vi "SLL DE DAQ Info Display.vi"(8 "error in (no error)":errorcluster) -> (0 "error out":errorcluster)   [LabVIEW 2013]
doc: "Copyright © 2005, Soliton Technologies.\nAll rights reserved."
uses:
  Controls/SLL DE DAQ Info Display Options.ctl
  Sub VIs/DAQ Engine/Controls/SLL DE DI Global Options.ctl
  Sub VIs/DAQ Engine/Controls/SLL DE Circular Buffer Options.ctl
  Sub VIs/DAQ Engine/Controls/SLL DE DO Global Options.ctl
  Sub VIs/DAQ Engine/Controls/SLL DE AO Global Options.ctl
  Sub VIs/DAQ Engine/Controls/SLL DE DAQ Global Options.ctl
  Sub VIs/DAQ Engine/Controls/SLL DE DAQ Global Elements.ctl
  Sub VIs/DAQ Engine/Controls/SLL DE List of Digital Inputs.ctl
  Sub VIs/DAQ Engine/Controls/SLL DE List of Analog Inputs.ctl
  Sub VIs/DAQ Engine/Controls/SLL DE List of Digital Outputs.ctl
  Sub VIs/DAQ Engine/Controls/SLL DE List of Analog Outputs.ctl
panel:
  in  "View File":bool
  in  "Virtual Chart":bool
  out "DO Running?":bool
  out "DI Running?":bool
  out "AO Running?":bool
  out "AI Running?":bool
  in  "List of Analog Outputs":T1
  in  "stop":bool
  in  "Tab Control":T2(tab)
  out "AI Status 3":cluster{"AI Value":sgl, "AI Name":string}[](array[cluster]) {"AI Value" format="%#.2f"}
  out "AI Status 2":cluster{"AI Value":sgl, "AI Name":string}[](array[cluster]) {"AI Value" format="%#.2f"}
  out "AI Status":cluster{"AI Value":sgl, "AI Name":string}[](array[cluster]) {"AI Value" format="%#.2f"}
  in  "AO Status":cluster{"AO Value":sgl, "AO Name":string}[](array[cluster]) {"AO Value" format="%#.2f"}
  in  "AO Status 2":cluster{"AO Value":sgl, "AO Name":string}[](array[cluster]) {"AO Value" format="%#.2f"}
  in  "AO Status 3":cluster{"AO Value":sgl, "AO Name":string}[](array[cluster]) {"AO Value" format="%#.2f"}
  out "DI Status 3":cluster{"DI Value?":bool, "DI Name":string}[](array[cluster])
  out "DI Status 2":cluster{"DI Value?":bool, "DI Name":string}[](array[cluster])
  out "DI Status":cluster{"DI Value?":bool, "DI Name":string}[](array[cluster])
  in  "DO Status 3":string[](array[string])
  in  "DO Value? 3":bool[](array[boolean]) caption="DO Value?"
  in  "DO Status 2":string[](array[string])
  in  "DO Value? 2":bool[](array[boolean]) caption="DO Value?"
  in  "DO Status":string[](array[string])
  in  "DO Value?":bool[](array[boolean]) caption="Enable Test"
  out "Date":string="Fri, Oct 10, 2003 3:32:43 AM"
  in  "List of Digital Outputs":T3=enum."STATION1_STOP TEST"
  in  "List of Analog Inputs":T4
  in  "List of Digital Inputs":T5
  # "<Project Name>"
  # "Logo"
  # "DAQ Info Display SCREEN"
  # "="
  # "="
  # "="
  # "-"
  # "-"
  # "-"
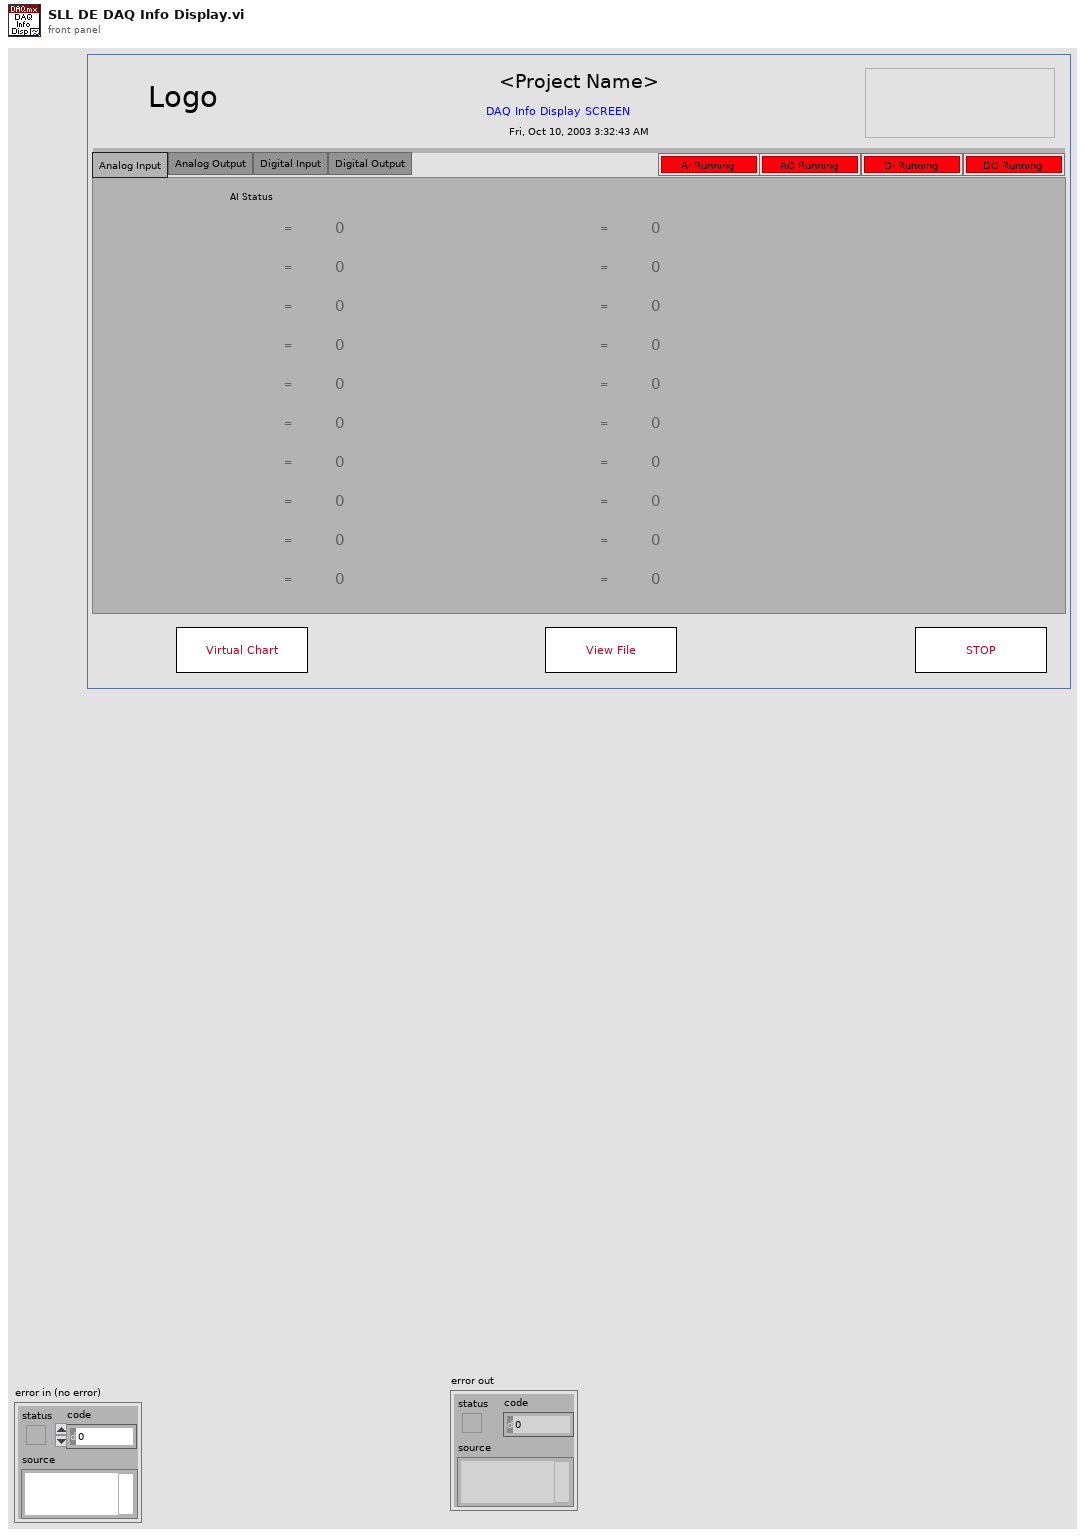
[diagram p1: front panel]
types:
  T1 = typedef "SLL DE List of Analog Outputs.ctl" = enum16{"None"}
  T2 = enum32{"Analog Input", "Analog Output", "Digital Input", "Digital Output"}
  T3 = typedef "SLL DE List of Digital Outputs.ctl" = enum16{"STATION1_START TEST", "STATION1_STOP TEST", "STATION1_LIGHT1", "STATION1_LIGHT2", "STATION1_LIGHT3", "STATION1_SELECT_TEST", "STATION2_START TEST", "STATION2_STOP TEST", "STATION2_LIGHT1", "STATION2_LIGHT2", "STATION2_LIGHT3", "STATION2_SELECT_TEST", "STATION3_START TEST", "STATION3_STOP TEST", "STATION3_LIGHT1", "STATION3_LIGHT2", "STATION3_LIGHT3", "STATION3_SELECT_TEST", "STATION4_START TEST", "STATION4_STOP TEST", "STATION4_LIGHT1", "STATION4_LIGHT2", "STATION4_LIGHT3", "STATION4_SELECT_TEST"}
  T4 = typedef "SLL DE List of Analog Inputs.ctl" = enum16{"None"}
  T5 = typedef "SLL DE List of Digital Inputs.ctl" = enum16{"STATION1_START", "STATION1_STOP", "STATION1_CLAMPED", "STATION1_TC_PASS", "STATION1_TC_FAIL", "STATION1_TTA", "STATION1_TTB", "STATION2_START", "STATION2_STOP", "STATION2_CLAMPED", "STATION2_TC_PASS", "STATION2_TC_FAIL", "STATION2_TTA", "STATION2_TTB", "STATION3_START", "STATION3_STOP", "STATION3_CLAMPED", "STATION3_TC_PASS", "STATION3_TC_FAIL", "STATION3_TTA", "STATION3_TTB", "STATION4_START", "STATION4_STOP", "STATION4_CLAMPED", "STATION4_TC_PASS", "STATION4_TC_FAIL", "STATION4_TTA", "STATION4_TTB"}
  T6 = typedef "SLL DE DAQ Info Display Options.ctl" = enum16{"Initialization", "Config AI/DI Controls", "Config AO Controls", "Config DO Controls", "Poll Events", "AI Read", "DI Read", "AO Write", "DO Write", "Launch Virtual Chart", "Launch File View", "Error", "Exit"}
  T7 = cluster{"DI Channel Names":string[], "DI Status":cluster{"DI ON?":bool, "DI Name":string}[], "AI Status":cluster{"AI Value":sgl, "AI Name":string}[], "DO Status":string[], "DO Value?":bool[], "AO Status":cluster{"AI Value":sgl, "AI Name":string}[]}
  T8 = typedef "SLL DE DO Global Options.ctl" = enum16{"Init", "Write Line", "Write Array", "Write Full Status", "Read Line", "Read Array", "Read Full Status", "Restart DO", "Send to Safe Mode", "Stop DO"}
  T9 = typedef "SLL DE AO Global Options.ctl" = enum16{"Init", "Write Line", "Write Array", "Read Line", "Read Array", "Read Full Status", "Restart AO", "Send to Safe Mode", "Stop AO"}
  T10 = typedef "SLL DE DAQ Global Options.ctl" = enum16{"Init", "Write 1", "Read 1", "Write Array", "Read Array", "Clear"}
  T11 = typedef "SLL DE Circular Buffer Options.ctl" = enum16{"Initialize", "Init Pointer X", "Write", "Read Single Value", "Read Pointer X (Multi Value)", "Clear Data"}
  T12 = typedef "SLL DE DI Global Options.ctl" = enum16{"Init", "Write Line", "Write Array", "Read Line", "Read Array", "Read Full Status", "Write Full Status"}
  T13 = typedef "SLL DE DAQ Global Elements.ctl" = enum16{"AI Error", "AO Error", "DI Error", "DO Error", "AI Restart", "DI Restart", "AI Running", "AO Running", "DI Running", "DO Running", "DAQ Exit?"}
  T14 = enum32{"Bad", "Idle", "Run top level", "Running"}
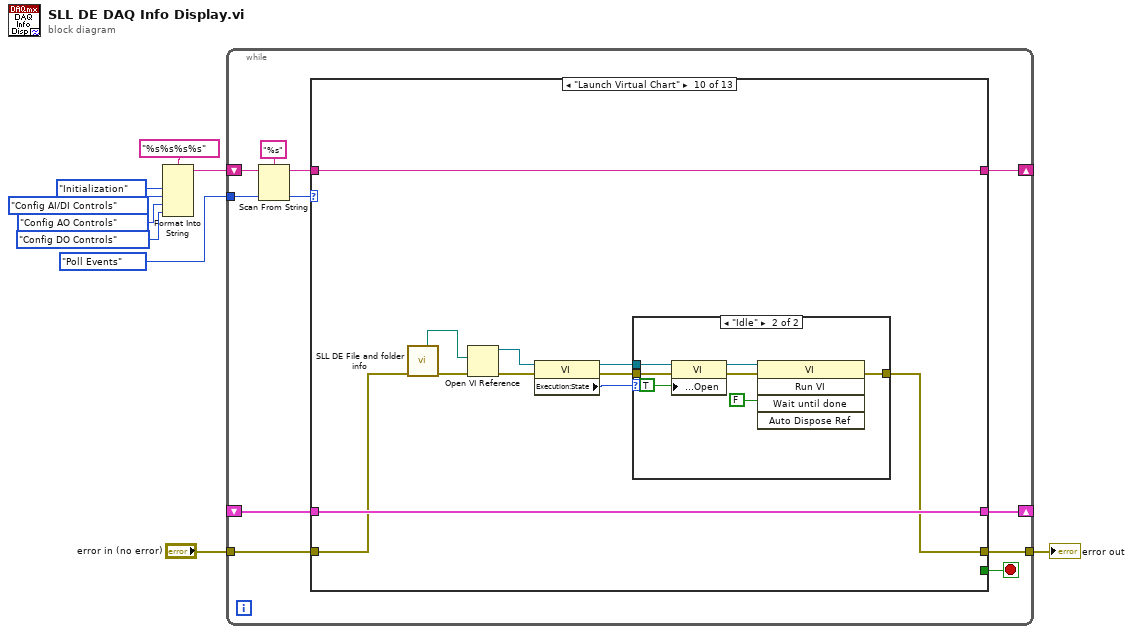
[diagram p0: block diagram]
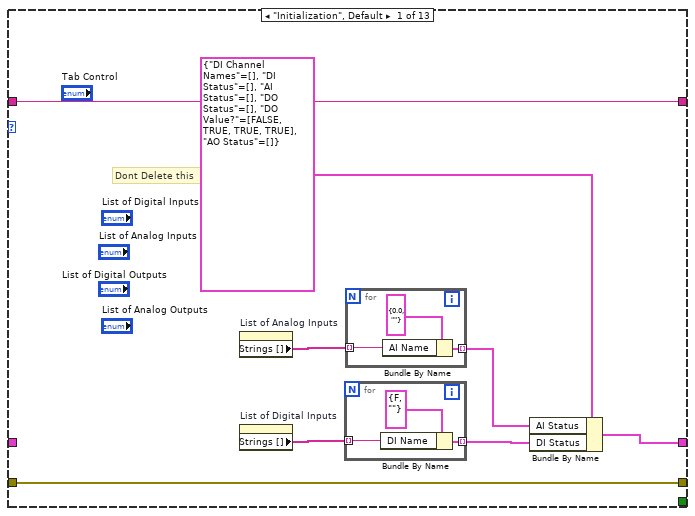
[diagram p2: hidden frame]
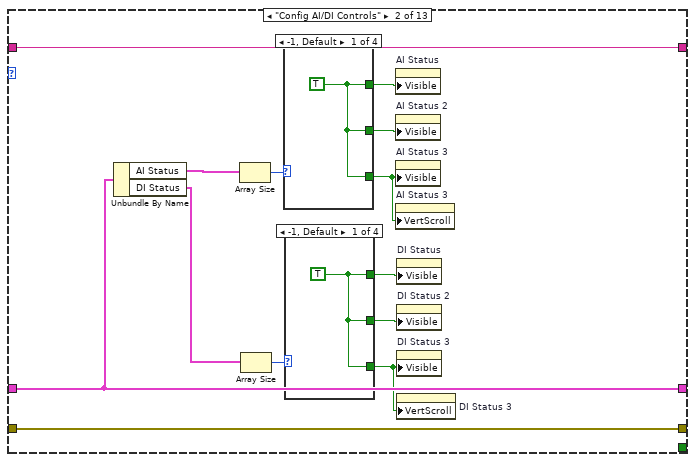
[diagram p3: hidden frame]
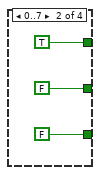
[diagram p4: hidden frame]
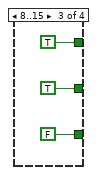
[diagram p5: hidden frame]
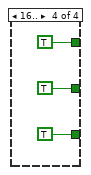
[diagram p6: hidden frame]
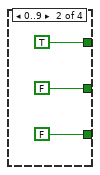
[diagram p7: hidden frame]
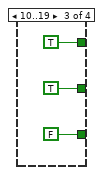
[diagram p8: hidden frame]
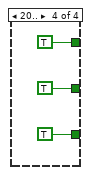
[diagram p9: hidden frame]
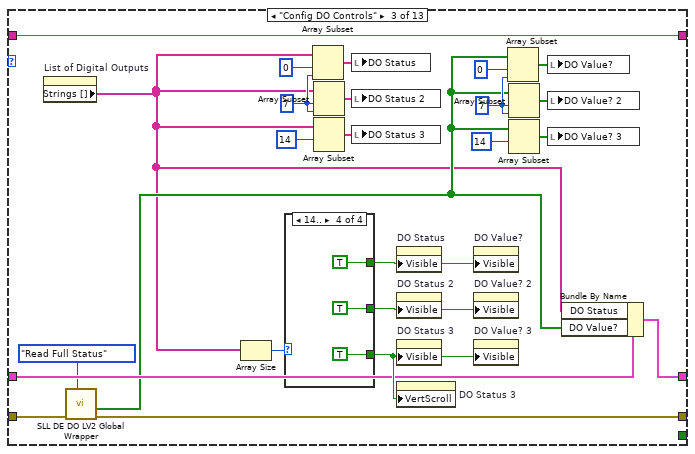
[diagram p10: hidden frame]
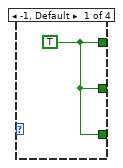
[diagram p11: hidden frame]
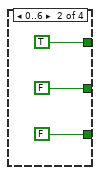
[diagram p12: hidden frame]
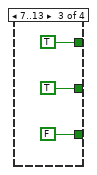
[diagram p13: hidden frame]
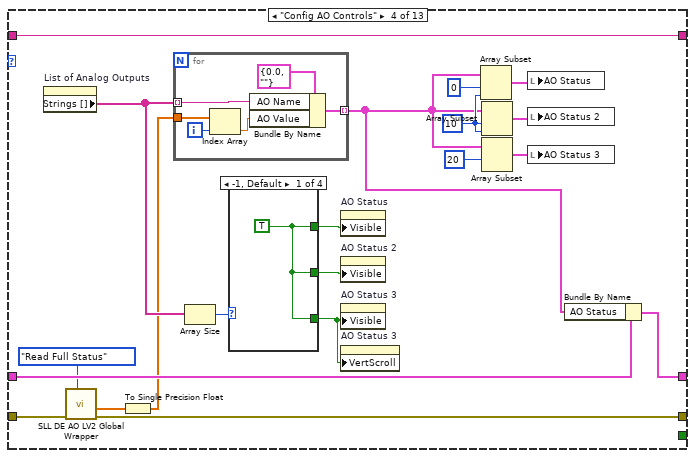
[diagram p14: hidden frame]
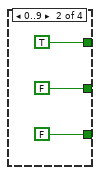
[diagram p15: hidden frame]
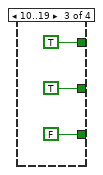
[diagram p16: hidden frame]
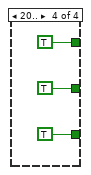
[diagram p17: hidden frame]
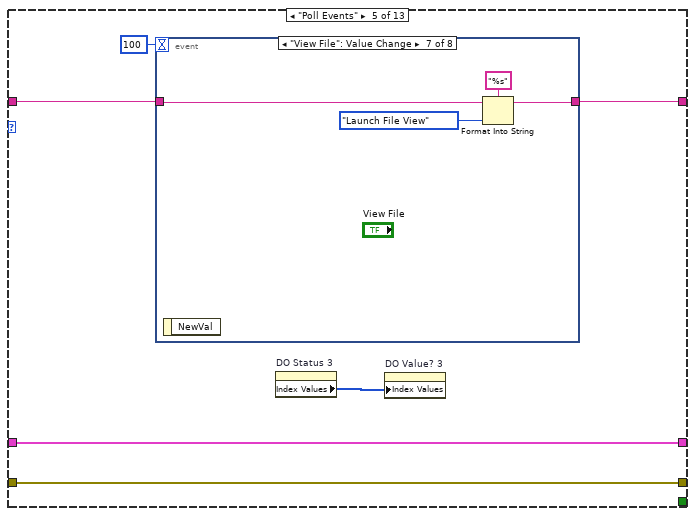
[diagram p18: hidden frame]
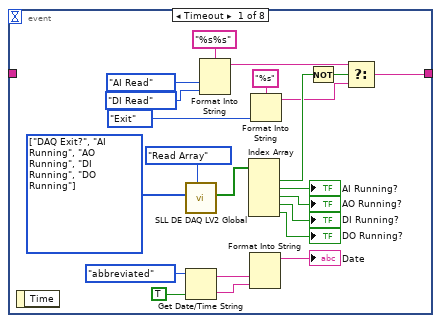
[diagram p19: hidden frame]
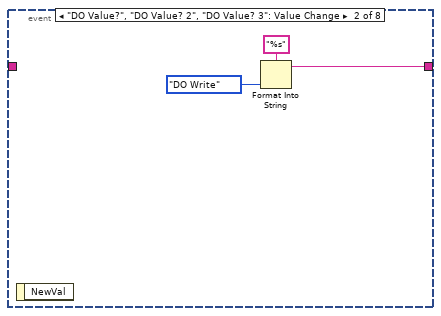
[diagram p20: hidden frame]
diagram:
  n1 = Format Into String(format string="%s%s%s%s", SLL_DE_DAQ_Info_Display_Options."Initialization" ("Case"), SLL_DE_DAQ_Info_Display_Options."Config AI/DI Controls" ("Case"), SLL_DE_DAQ_Info_Display_Options."Config AO Controls" ("Case"), SLL_DE_DAQ_Info_Display_Options."Config DO Controls" ("Case")) -> (resulting string=w8:string)  [unwired: 2 in, 1 out]
  n2 = while {
    shift-right: [w16] -> _
    shift-left: w8 -> [w20]
    tunnel: SLL_DE_DAQ_Info_Display_Options."Poll Events" ("Case") -> [w18]
    tunnel: [w14] -> w5
    tunnel: "error in (no error)" -> [w13]
    shift-right: [w11] -> _
    shift-left: _ -> [w10]
    stop <- w12 stop-if-true
    n3 = Scan From String(format string="%s", input string=w20, default 1=w18) -> (remaining string=w15:string, output 1=w17:T6)  [unwired: 2 in, 2 out]
    n4 = case shown="\"Launch Virtual Chart\"" w17 {
      tunnel: [w28 w44 w91 w121 w140 w229 w250 w270 w297 w308 w327 w338 w342] -> w16
      tunnel: w15 -> [w28 w44 w91 w121 w141 w229 w250 w270 w297 w308 w327 w338 w342]
      tunnel: [w21 w46 w76 w108 w143 w224 w248 w260 w293 w298 w318 w337 w341] -> w14
      tunnel: w13 -> [w21 w46 w77 w109 w143 w225 w249 w261 w294 w306 w325 w337 w341]
      tunnel: [_ _ _ _ _ _ _ _ _ _ _ _ TRUE] -> w12
      tunnel: [w25 w45 w85 w115 w142 w226 w246 w269 w296 w307 w326 w336 w339] -> w11
      tunnel: w10 -> [_ w45 w86 w116 w142 w226 w246 w269 w296 w307 w326 w336 w339]
      frame "Initialization", Default {
        # "Dont Delete this"
        n5 = property on="List of Analog Inputs" class="Enum (strict)"() -> ("Strings []"=w22:string[])  [unwired: 2 in, 2 out]
        n6 = property on="List of Digital Inputs" class="Enum (strict)"() -> ("Strings []"=w27:string[])  [unwired: 2 in, 2 out]
        n7 = for {
          tunnel: w27 -> [w33] mode=indexing
          tunnel: [w32] -> w24 mode=indexing
          n8 = Bundle By Name(cluster=cluster{"DI ON?":bool, "DI Name":string} {"DI ON?"=FALSE, "DI Name"=""} ("Filter Status 2"), "DI Name"=w33) -> (w32:cluster{"DI ON?":bool, "DI Name":string})
        }
        n9 = for {
          tunnel: w22 -> [w31] mode=indexing
          tunnel: [w30] -> w23 mode=indexing
          n10 = Bundle By Name(cluster=cluster{"AI Value":sgl, "AI Name":string} {"AI Value"=0.0, "AI Name"=""} ("Filter Status 2"), "AI Name"=w31) -> (w30:cluster{"AI Value":sgl, "AI Name":string})
        }
        n11 = Bundle By Name(cluster=T7 {"DI Channel Names"=[], "DI Status"=[], "AI Status"=[], "DO Status"=[], "DO Value?"=[FALSE, TRUE, TRUE, TRUE], "AO Status"=[]}, "AI Status"=w23, "DI Status"=w24) -> (w25:T7)
      }
      frame "Config AI/DI Controls" {
        n12 = Unbundle By Name(w45) -> ("AI Status"=w47:cluster{"AI Value":sgl, "AI Name":string}[], "DI Status"=w35:cluster{"DI ON?":bool, "DI Name":string}[])
        n13 = Array Size(array=w47) -> (size(s)=w43:i32)
        n14 = Array Size(array=w35) -> (size(s)=w36:i32)
        n15 = case shown="-1, Default" w43 {
          tunnel: [w58 TRUE ("Visible") TRUE ("Visible") TRUE ("Visible")] -> w42
          tunnel: [w58 FALSE ("Visible") TRUE ("Visible") TRUE ("Visible")] -> w41
          tunnel: [w58 FALSE ("Visible") FALSE ("Visible") TRUE ("Visible")] -> w40
          frame -1, Default {
            w58 = TRUE ("Visible")
          }
          frame 0..9 {
          }
          frame 10..19 {
          }
          frame 20.. {
          }
        }
        n16 = case shown="-1, Default" w36 {
          tunnel: [w48 TRUE ("Visible") TRUE ("Visible") TRUE ("Visible")] -> w37
          tunnel: [w48 FALSE ("Visible") TRUE ("Visible") TRUE ("Visible")] -> w38
          tunnel: [w48 FALSE ("Visible") FALSE ("Visible") TRUE ("Visible")] -> w39
          frame -1, Default {
            w48 = TRUE ("Visible")
          }
          frame 0..7 {
          }
          frame 8..15 {
          }
          frame 16.. {
          }
        }
        n17 = property on="AI Status" class="Arr (strict)"("Visible"=w42) -> ()  [unwired: 2 in, 2 out]
        n18 = property on="AI Status 2" class="Arr (strict)"("Visible"=w41) -> ()  [unwired: 2 in, 2 out]
        n19 = property on="AI Status 3" class="Arr (strict)"("Visible"=w40) -> ()  [unwired: 2 in, 2 out]
        n20 = property on="AI Status 3" class="Arr (strict)"("VertScroll"=w40) -> ()  [unwired: 2 in, 2 out]
        n21 = property on="DI Status" class="Arr (strict)"("Visible"=w37) -> ()  [unwired: 2 in, 2 out]
        n22 = property on="DI Status 2" class="Arr (strict)"("Visible"=w38) -> ()  [unwired: 2 in, 2 out]
        n23 = property on="DI Status 3" class="Arr (strict)"("Visible"=w39) -> ()  [unwired: 2 in, 2 out]
        n24 = property on="DI Status 3" class="Arr (strict)"("VertScroll"=w39) -> ()  [unwired: 2 in, 2 out]
      }
      frame "Config DO Controls" {
        w74 = 7 ("length")
        w83 = 7 ("length")
        n25 = property on="List of Digital Outputs" class="Enum (strict)"() -> ("Strings []"=w68:string[])  [unwired: 2 in, 2 out]
        n26 = call "SLL DE DO LV2 Global Wrapper.vi"("DO Option"=SLL_DE_DO_Global_Options."Read Full Status", "error in (no error)"=w77) -> ("error out"=w76:errorcluster, "Digital Output Array Value"=w69:bool[])  [unwired: 6 in, 2 out]
        n27 = Array Size(array=w68) -> (size(s)=w90:i32)
        n28 = case shown="14.." w90 {
          tunnel: [w92 TRUE ("Visible") TRUE ("Visible") TRUE ("Visible")] -> w87
          tunnel: [w92 FALSE ("Visible") TRUE ("Visible") TRUE ("Visible")] -> w88
          tunnel: [w92 FALSE ("Visible") FALSE ("Visible") TRUE ("Visible")] -> w89
          frame -1, Default {
            w92 = TRUE ("Visible")
          }
          frame 0..6 {
          }
          frame 7..13 {
          }
          frame 14.. {
          }
        }
        n29 = Array Subset(array=w68, index=0, length=w83) -> (w81:string[])
        n30 = Array Subset(array=w68, index=w83, length=w83) -> (w80:string[])
        n31 = Array Subset(array=w68, index=14) -> (w79:string[])  [unwired: 1 in]
        n32 = local write "DO Status"(w81) -> ()
        n33 = local write "DO Status 2"(w80) -> ()
        n34 = local write "DO Status 3"(w79) -> ()
        n35 = property on="DO Status" class="Arr (strict)"("Visible"=w87) -> ()  [unwired: 2 in, 2 out]
        n36 = property on="DO Status 2" class="Arr (strict)"("Visible"=w88) -> ()  [unwired: 2 in, 2 out]
        n37 = property on="DO Status 3" class="Arr (strict)"("Visible"=w89) -> ()  [unwired: 2 in, 2 out]
        n38 = property on="DO Status 3" class="Arr (strict)"("VertScroll"=w89) -> ()  [unwired: 2 in, 2 out]
        n39 = property on="DO Value?" class="Arr (strict)"("Visible"=w87) -> ()  [unwired: 2 in, 2 out]
        n40 = property on="DO Value? 2" class="Arr (strict)"("Visible"=w88) -> ()  [unwired: 2 in, 2 out]
        n41 = property on="DO Value? 3" class="Arr (strict)"("Visible"=w89) -> ()  [unwired: 2 in, 2 out]
        n42 = Array Subset(array=w69, index=0, length=w74) -> (w72:bool[])
        n43 = Array Subset(array=w69, index=w74, length=w74) -> (w71:bool[])
        n44 = Array Subset(array=w69, index=14) -> (w70:bool[])  [unwired: 1 in]
        n45 = local write "DO Value?"(w72) -> ()
        n46 = local write "DO Value? 2"(w71) -> ()
        n47 = local write "DO Value? 3"(w70) -> ()
        n48 = Bundle By Name(cluster=w86, "DO Status"=w68, "DO Value?"=w69) -> (w85:T7)
      }
      frame "Config AO Controls" {
        w113 = 10 ("length")
        n49 = property on="List of Analog Outputs" class="Enum (strict)"() -> ("Strings []"=w111:string[])  [unwired: 2 in, 2 out]
        n50 = call "SLL DE AO LV2 Global Wrapper.vi"("AO Option"=SLL_DE_AO_Global_Options."Read Full Status", "error in (no error)"=w109) -> ("error out"=w108:errorcluster, "Analog Output Array Value"=w106:dbl[])  [unwired: 6 in, 2 out]
        n51 = To Single Precision Float(number=w106) -> (single precision float=w102:sgl[])
        n52 = for {
          tunnel: w111 -> [w127] mode=indexing
          tunnel: [w126] -> w110 mode=indexing
          tunnel: w102 -> [w124]
          i -> [w122]
          n53 = Index Array(array=w124, index=w122) -> (element=w123:sgl)
          n54 = Bundle By Name(cluster=cluster{"AO Value":sgl, "AO Name":string} {"AO Value"=0.0, "AO Name"=""} ("Filter Status 2"), "AO Name"=w127, "AO Value"=w123) -> (w126:cluster{"AO Value":sgl, "AO Name":string})
        }
        n55 = Array Size(array=w111) -> (size(s)=w120:i32)
        n56 = case shown="-1, Default" w120 {
          tunnel: [w128 TRUE ("Visible") TRUE ("Visible") TRUE ("Visible")] -> w117
          tunnel: [w128 FALSE ("Visible") TRUE ("Visible") TRUE ("Visible")] -> w118
          tunnel: [w128 FALSE ("Visible") FALSE ("Visible") TRUE ("Visible")] -> w119
          frame -1, Default {
            w128 = TRUE ("Visible")
          }
          frame 0..9 {
          }
          frame 10..19 {
          }
          frame 20.. {
          }
        }
        n57 = property on="AO Status" class="Arr (strict)"("Visible"=w117) -> ()  [unwired: 2 in, 2 out]
        n58 = property on="AO Status 2" class="Arr (strict)"("Visible"=w118) -> ()  [unwired: 2 in, 2 out]
        n59 = property on="AO Status 3" class="Arr (strict)"("Visible"=w119) -> ()  [unwired: 2 in, 2 out]
        n60 = property on="AO Status 3" class="Arr (strict)"("VertScroll"=w119) -> ()  [unwired: 2 in, 2 out]
        n61 = Array Subset(array=w110, index=0, length=w113) -> (w105:cluster{"AO Value":sgl, "AO Name":string}[])
        n62 = Array Subset(array=w110, index=w113, length=w113) -> (w104:cluster{"AO Value":sgl, "AO Name":string}[])
        n63 = Array Subset(array=w110, index=20) -> (w103:cluster{"AO Value":sgl, "AO Name":string}[])  [unwired: 1 in]
        n64 = local write "AO Status"(w105) -> ()
        n65 = local write "AO Status 2"(w104) -> ()
        n66 = local write "AO Status 3"(w103) -> ()
        n67 = Bundle By Name(cluster=w116, "AO Status"=w110) -> (w115:T7)
      }
      frame "Poll Events" {
        n68 = event shown="[6] \"View File\": Value Change" {
          selector: _ -> [_ _ _ _ _ _ _ _]
          dyn-events: _ -> [_ _ _ _ _ _ _ _]
          timeout: 100 -> [_ _ _ _ _ _ _ _]
          tunnel: w141 -> [_ _ w174 w186 w198 w205 w209 _]
          tunnel: [w148 w166 w175 w187 w199 w206 w210 w213] -> w140
          event Timeout {
            w156 = T13[] [enum."DAQ Exit?", enum."AI Running", enum."AO Running", enum."DI Running", enum."DO Running"] items=["AI Error", "AO Error", "DI Error", "DO Error", "AI Restart", "DI Restart", "AI Running", "AO Running", "DI Running", "DO Running", "DAQ Exit?"] ("Elements Array")
            n69 = event-data() -> ()  [unwired: 1 in, 1 out]
            n70 = call "SLL DE DAQ LV2 Global.vi"("Option"=SLL_DE_DAQ_Global_Options."Read Array", "Elements Array"=w156) -> ("Status Array Out"=w155:bool[])  [unwired: 7 in, 2 out]
            n71 = Get Date/Time String(date format (0)=enum16{"short", "long", "abbreviated"}."abbreviated", want seconds? (F)=TRUE) -> (date string=w160:string, time string=w159:string)  [unwired: 1 in]
            n72 = Format Into String(format string="%s%s", SLL_DE_DAQ_Info_Display_Options."AI Read" ("Case"), SLL_DE_DAQ_Info_Display_Options."DI Read" ("Case")) -> (resulting string=w149:string)  [unwired: 2 in, 1 out]
            n73 = Index Array(array=w155) -> (element #1=w150:bool, element #2=→"AI Running?":bool, element #3=→"AO Running?":bool, element #4=→"DI Running?":bool, element #5=→"DO Running?":bool)  [unwired: 5 in]
            n74 = Format Into String(w160, w159) -> (resulting string=→"Date":string)  [unwired: 3 in, 1 out]
            n75 = Format Into String(format string="%s", SLL_DE_DAQ_Info_Display_Options."Exit" ("Case")) -> (resulting string=w145:string)  [unwired: 2 in, 1 out]
            n76 = Not(x=w150) -> (.not. x?=w144:bool)
            n77 = Select(t=w149, s=w144, f=w145) -> (s? t:f=w148:string)
          }
          event "DO Value?", "DO Value? 2", "DO Value? 3": Value Change {
            n78 = event-data() -> ()  [unwired: 1 in, 1 out]
            n79 = Format Into String(format string="%s", SLL_DE_DAQ_Info_Display_Options."DO Write" ("Case")) -> (resulting string=w166:string)  [unwired: 2 in, 1 out]
          }
          event "AO Status": Value Change {
            n80 = event-data() -> ("NewVal"=w173:cluster{"AO Value":sgl, "AO Name":string}[], "OldVal"=w172:cluster{"AO Value":sgl, "AO Name":string}[])  [unwired: 1 in]
            n81 = Array Size(array=w173) -> (size(s)=w171:i32)
            n82 = Array Size(array=w172) -> (size(s)=w169:i32)
            n83 = Not Equal?(x=w171, y=w169) -> (x != y?=w170:bool)
            n84 = case shown="True" w170 {
              tunnel: w169 -> [_ w178]
              frame False {
              }
              frame True {
                n85 = local read "AO Status"() -> (w180:cluster{"AO Value":sgl, "AO Name":string}[])
                n86 = Split 1D Array(array=w180, index=w178) -> (first subarray=w179:cluster{"AO Value":sgl, "AO Name":string}[])  [unwired: 1 out]
                n87 = local write "AO Status"(w179) -> ()
              }
            }
            n88 = Format Into String(format string="%s", initial string=w174, SLL_DE_DAQ_Info_Display_Options."AO Write" ("Case")) -> (resulting string=w175:string)  [unwired: 1 in, 1 out]
          }
          event "AO Status 2": Value Change {
            n89 = event-data() -> ("NewVal"=w185:cluster{"AO Value":sgl, "AO Name":string}[], "OldVal"=w184:cluster{"AO Value":sgl, "AO Name":string}[])  [unwired: 1 in]
            n90 = Array Size(array=w185) -> (size(s)=w183:i32)
            n91 = Array Size(array=w184) -> (size(s)=w181:i32)
            n92 = Not Equal?(x=w183, y=w181) -> (x != y?=w182:bool)
            n93 = case shown="True" w182 {
              tunnel: w181 -> [_ w190]
              frame False {
              }
              frame True {
                n94 = local read "AO Status 2"() -> (w192:cluster{"AO Value":sgl, "AO Name":string}[])
                n95 = Split 1D Array(array=w192, index=w190) -> (first subarray=w191:cluster{"AO Value":sgl, "AO Name":string}[])  [unwired: 1 out]
                n96 = local write "AO Status 2"(w191) -> ()
              }
            }
            n97 = Format Into String(format string="%s", initial string=w186, SLL_DE_DAQ_Info_Display_Options."AO Write" ("Case")) -> (resulting string=w187:string)  [unwired: 1 in, 1 out]
          }
          event "AO Status 3": Value Change {
            n98 = event-data() -> ("NewVal"=w197:cluster{"AO Value":sgl, "AO Name":string}[], "OldVal"=w196:cluster{"AO Value":sgl, "AO Name":string}[])  [unwired: 1 in]
            n99 = Array Size(array=w197) -> (size(s)=w195:i32)
            n100 = Array Size(array=w196) -> (size(s)=w193:i32)
            n101 = Not Equal?(x=w195, y=w193) -> (x != y?=w194:bool)
            n102 = case shown="True" w194 {
              tunnel: w193 -> [_ w202]
              frame False {
              }
              frame True {
                n103 = local read "AO Status 3"() -> (w204:cluster{"AO Value":sgl, "AO Name":string}[])
                n104 = Split 1D Array(array=w204, index=w202) -> (first subarray=w203:cluster{"AO Value":sgl, "AO Name":string}[])  [unwired: 1 out]
                n105 = local write "AO Status 3"(w203) -> ()
              }
            }
            n106 = Format Into String(format string="%s", initial string=w198, SLL_DE_DAQ_Info_Display_Options."AO Write" ("Case")) -> (resulting string=w199:string)  [unwired: 1 in, 1 out]
          }
          event "Virtual Chart": Value Change {
            n107 = event-data() -> ()  [unwired: 1 in, 1 out]
            n108 = Format Into String(format string="%s", initial string=w205, SLL_DE_DAQ_Info_Display_Options."Launch Virtual Chart" ("Case")) -> (resulting string=w206:string)  [unwired: 1 in, 1 out]
          }
          event "View File": Value Change {
            n109 = event-data() -> ()  [unwired: 1 in, 1 out]
            n110 = Format Into String(format string="%s", initial string=w209, SLL_DE_DAQ_Info_Display_Options."Launch File View" ("Case")) -> (resulting string=w210:string)  [unwired: 1 in, 1 out]
          }
          event "stop": Value Change {
            n111 = event-data() -> ()  [unwired: 1 in, 1 out]
            n112 = Format Into String(format string="%s", SLL_DE_DAQ_Info_Display_Options."Exit" ("Case")) -> (resulting string=w213:string)  [unwired: 2 in, 1 out]
          }
        }
        n113 = property on="DO Status 3" class="Arr (strict)"() -> ("Index Values"=w138:u32[])  [unwired: 2 in, 2 out]
        n114 = property on="DO Value? 3" class="Arr (strict)"("Index Values"=w138) -> ()  [unwired: 2 in, 2 out]
      }
      frame "AI Read" {
        w221 = 10 ("length")
        n115 = Unbundle By Name(w226) -> ("AI Status"=w227:cluster{"AI Value":sgl, "AI Name":string}[])
        n116 = call "SLL DE AI Circular Buffer.vi"("Options"=SLL_DE_Circular_Buffer_Options."Read Single Value", "error in (no error)"=w225) -> ("error Out"=w224:errorcluster, "Output points"=w228:sgl[])  [unwired: 4 in, 4 out]
        n117 = for {
          shift-right: [w231] -> w218
          shift-left: w227 -> [w233]
          tunnel: w228 -> [w230] mode=indexing
          i -> [w232]
          n118 = in-place {
            in-place-border: w230 -> [w234]
            n119 = in-place-array #1(w233, w232) -> (w236:cluster{"AI Value":sgl, "AI Name":string})
            n120 = Bundle By Name(cluster=w236, "AI Value"=w234) -> (w235:cluster{"AI Value":sgl, "AI Name":string})
            n121 = in-place-array #1(w235) -> (w231:cluster{"AI Value":sgl, "AI Name":string}[])  [unwired: 1 out]
          }
        }
        n122 = Array Subset(array=w218, index=0, length=w221) -> (→"AI Status":cluster{"AI Value":sgl, "AI Name":string}[])
        n123 = Array Subset(array=w218, index=w221, length=w221) -> (→"AI Status 2":cluster{"AI Value":sgl, "AI Name":string}[])
        n124 = Array Subset(array=w218, index=20) -> (→"AI Status 3":cluster{"AI Value":sgl, "AI Name":string}[])  [unwired: 1 in]
      }
      frame "DI Read" {
        w242 = 8 ("length")
        n125 = Unbundle By Name(w246) -> ("DI Status"=w245:cluster{"DI ON?":bool, "DI Name":string}[])
        n126 = call "SLL DE DI LV2 Global.vi"("Option"=SLL_DE_DI_Global_Options."Read Full Status", "error in (no error)"=w249) -> ("error out"=w248:errorcluster, "Digital Array Status"=w244:bool[])  [unwired: 6 in, 2 out]
        n127 = for {
          shift-right: [w252] -> w240
          shift-left: w245 -> [w254]
          tunnel: w244 -> [w251] mode=indexing
          i -> [w253]
          n128 = in-place {
            in-place-border: w251 -> [w255]
            n129 = in-place-array #2(w254, w253) -> (w257:cluster{"DI ON?":bool, "DI Name":string})
            n130 = Bundle By Name(cluster=w257, "DI ON?"=w255) -> (w256:cluster{"DI ON?":bool, "DI Name":string})
            n131 = in-place-array #2(w256) -> (w252:cluster{"DI ON?":bool, "DI Name":string}[])  [unwired: 1 out]
          }
        }
        n132 = Array Subset(array=w240, index=0, length=w242) -> (→"DI Status":cluster{"DI ON?":bool, "DI Name":string}[])
        n133 = Array Subset(array=w240, index=w242, length=w242) -> (→"DI Status 2":cluster{"DI ON?":bool, "DI Name":string}[])
        n134 = Array Subset(array=w240, index=16) -> (→"DI Status 3":cluster{"DI ON?":bool, "DI Name":string}[])  [unwired: 1 in]
      }
      frame "AO Write" {
        n135 = for {
          tunnel: "AO Status 3" -> [w272] mode=indexing
          tunnel: [w271] -> w263 mode=indexing
          n136 = Unbundle By Name(w272) -> ("AO Value"=w271:sgl)
        }
        n137 = for {
          tunnel: "AO Status 2" -> [w274] mode=indexing
          tunnel: [w273] -> w264 mode=indexing
          n138 = Unbundle By Name(w274) -> ("AO Value"=w273:sgl)
        }
        n139 = for {
          tunnel: "AO Status" -> [w276] mode=indexing
          tunnel: [w275] -> w265 mode=indexing
          n140 = Unbundle By Name(w276) -> ("AO Value"=w275:sgl)
        }
        n141 = Build Array (concatenate)(w265, w264, w263) -> (w259:sgl[])
        n142 = To Double Precision Float(number=w259) -> (double precision float=w258:dbl[])
        n143 = call "SLL DE AO LV2 Global Wrapper.vi"("AO value Array"=w258, "AO Option"=SLL_DE_AO_Global_Options."Read Full Status", "error in (no error)"=w261) -> ("error out"=w260:errorcluster)  [unwired: 5 in, 3 out]
      }
      frame "DO Write" {
        n144 = Array Size(array="DO Status") -> (size(s)=w282:i32)
        n145 = Array Size(array="DO Status 2") -> (size(s)=w285:i32)
        n146 = Array Size(array="DO Status 3") -> (size(s)=w292:i32)
        n147 = Array Subset(array="DO Value?", index=0, length=w282) -> (w277:bool[])
        n148 = Array Subset(array="DO Value? 2", index=0, length=w285) -> (w278:bool[])
        n149 = Array Subset(array="DO Value? 3", index=0, length=w292) -> (w288:bool[])
        n150 = local write "DO Value?"(w277) -> ()
        n151 = local write "DO Value? 2"(w278) -> ()
        n152 = local write "DO Value? 3"(w288) -> ()
        n153 = Build Array (concatenate)(w277, w278, w288) -> (w287:bool[])
        n154 = call "SLL DE DO LV2 Global Wrapper.vi"("DO value Array"=w287, "DO Option"=SLL_DE_DO_Global_Options."Write Full Status", "error in (no error)"=w294) -> ("error out"=w293:errorcluster)  [unwired: 5 in, 3 out]
      }
      frame "Launch Virtual Chart" {
        n155 = call "SLL DE File and folder info.vi"("error in (no error)"=w306) -> ("error out"=w299:errorcluster, "Virtual Chart"=w300:path)  [unwired: 5 in, 4 out]
        n156 = Open VI Reference(vi path=w300, error in (no error)=w299) -> (vi reference=w301:refnum<vi>, error out=w302:errorcluster)  [unwired: 4 in]
        n157 = property class="VI"(reference=w301, error in=w302) -> (reference out=w303:refnum<vi>, error out=w304:errorcluster, "Execution:State"=w305:T14)
        n158 = case shown="\"Idle\"" w305 {
          tunnel: [w309 w312] -> w298
          tunnel: w303 -> [_ w314]
          tunnel: w304 -> [w309 w313]
          frame "Bad", Default {
          }
          frame "Idle" {
            n159 = property class="VI"(reference=w314, error in=w313, "Front Panel Window:Open"=TRUE) -> (reference out=w316:refnum<vi>, error out=w315:errorcluster)
            n160 = invoke class="VI" method="Run VI"(reference=w316, error in=w315, "Wait until done"=FALSE ("Wait Until Done")) -> (error out=w312:errorcluster)  [unwired: 2 in, 4 out]
          }
        }
      }
      frame "Launch File View" {
        n161 = call "SLL DE File and folder info.vi"("error in (no error)"=w325) -> ("error out"=w319:errorcluster, "View File"=w317:path)  [unwired: 5 in, 4 out]
        n162 = Open VI Reference(vi path=w317, error in (no error)=w319) -> (vi reference=w320:refnum<vi>, error out=w321:errorcluster)  [unwired: 4 in]
        n163 = property class="VI"(reference=w320, error in=w321) -> (reference out=w322:refnum<vi>, error out=w323:errorcluster, "Execution:State"=w324:T14)
        n164 = case shown="\"Idle\"" w324 {
          tunnel: [w328 w331] -> w318
          tunnel: w322 -> [_ w333]
          tunnel: w323 -> [w328 w332]
          frame "Bad", Default {
          }
          frame "Idle" {
            n165 = property class="VI"(reference=w333, error in=w332, "Front Panel Window:Open"=TRUE) -> (reference out=w335:refnum<vi>, error out=w334:errorcluster)
            n166 = invoke class="VI" method="Run VI"(reference=w335, error in=w334, "Wait until done"=FALSE ("Wait Until Done")) -> (error out=w331:errorcluster)  [unwired: 2 in, 4 out]
          }
        }
      }
      frame "Error" {
      }
      frame "Exit" {
      }
    }
  }
  "error out" <- w5
